vi "SaveSpe.vi"(0 "Live Time":dbl=1000.0, 1 "Z":dbl, 2 "Y":dbl, 3 "X":dbl, 4 "Real Time":dbl=1000.0, 5 "Spectrum":i32[](array[numeric]), 6 "name":string, 7 "data folder path":path) -> ()   [LabVIEW 2015]
panel:
  out "data size":i32
  out "error out 2":errorcluster
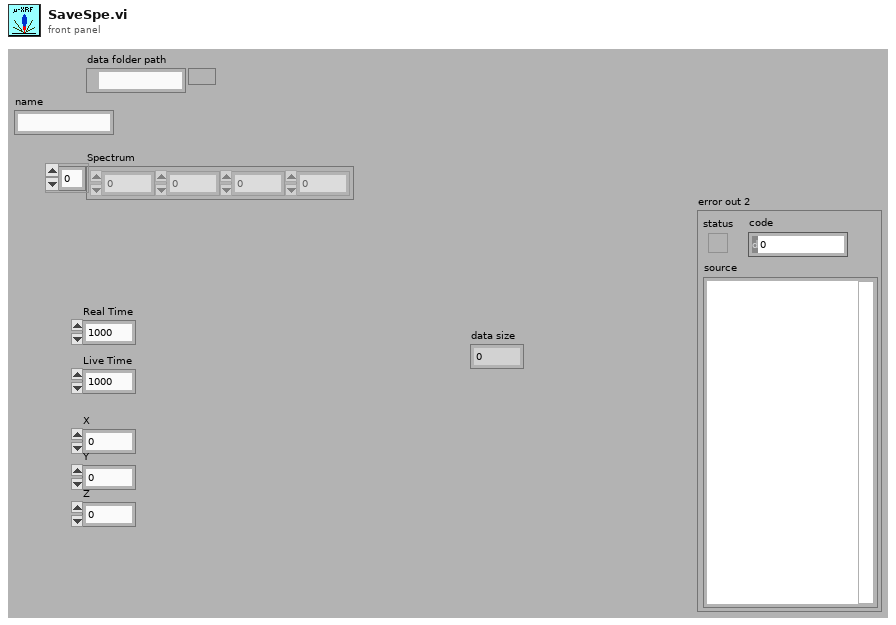
[diagram p1: front panel]
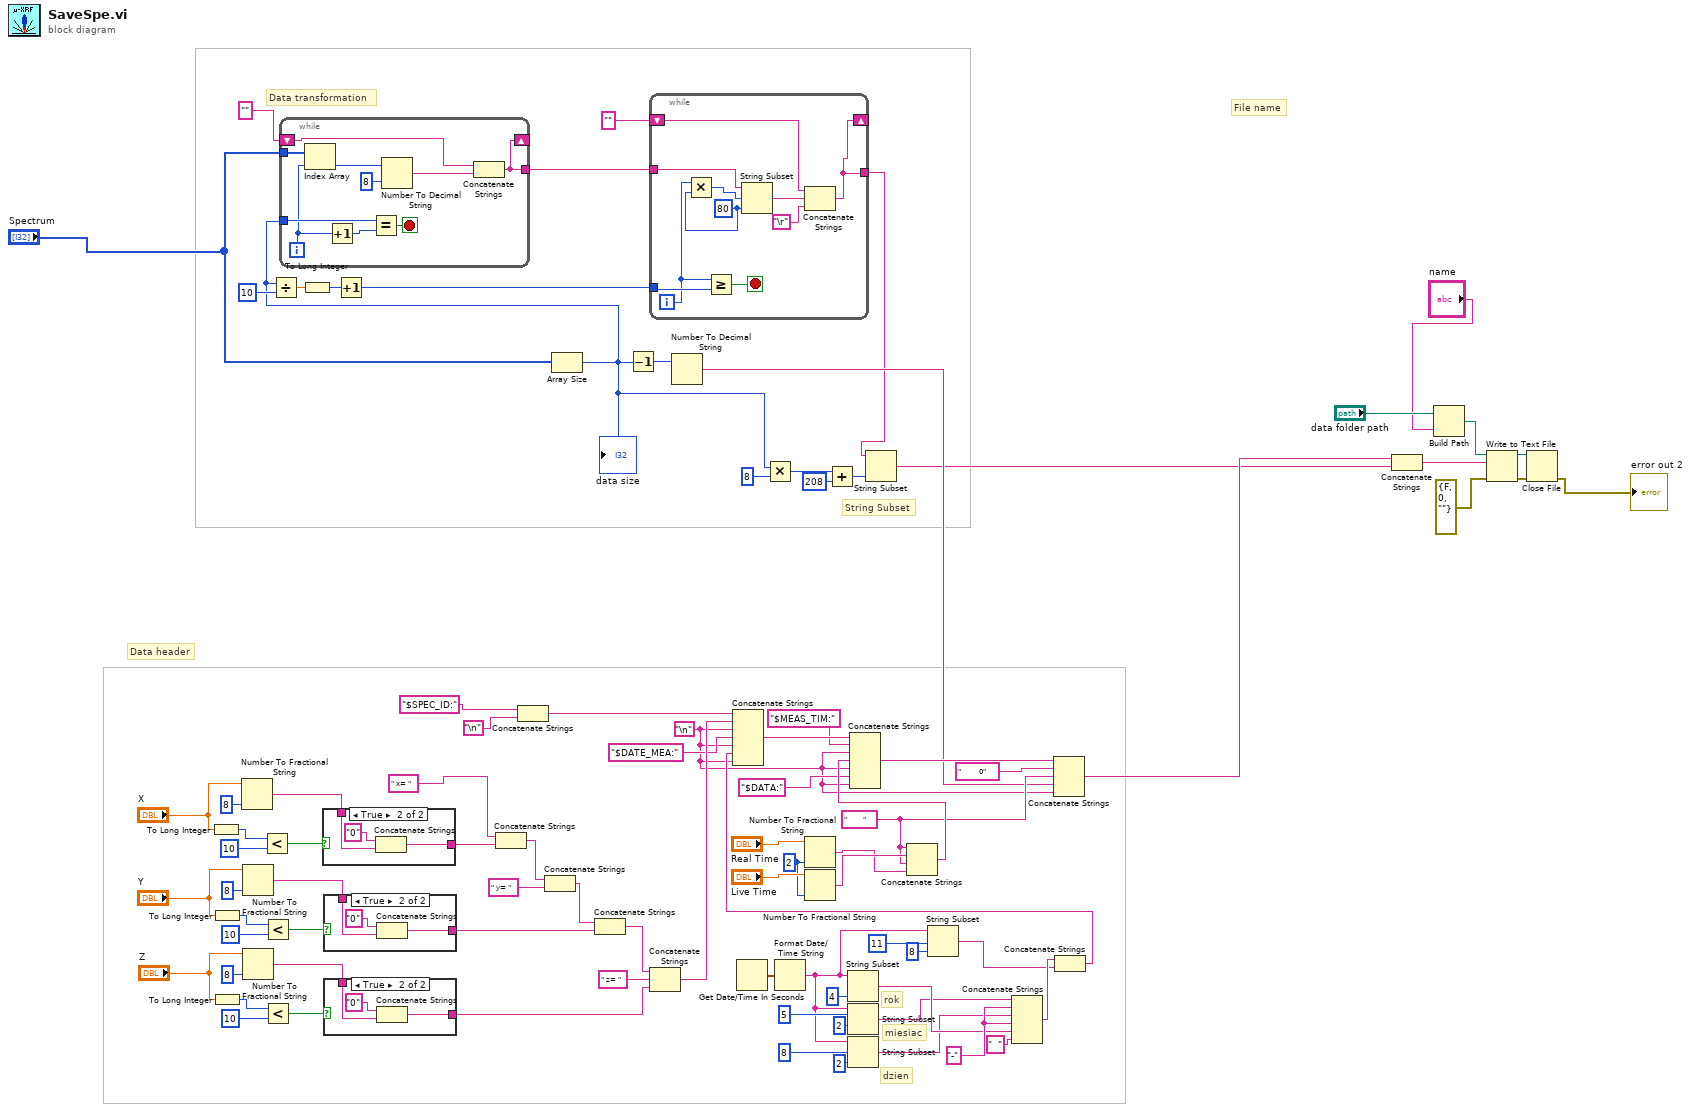
[diagram p0: block diagram]
diagram:
  w4 = i16 2 ("precision (6)")
  w29 = "        "
  w51 = "-"
  w27 = "\n"
  # "String Subset"
  # "Data transformation"
  # "Data header"
  # "File name"
  # "dzien"
  # "miesiac"
  # "rok"
  n1 = To Long Integer(number="X") -> (32bit integer=w83:i32)
  n2 = To Long Integer(number="Y") -> (32bit integer=w76:i32)
  n3 = To Long Integer(number="Z") -> (32bit integer=w69:i32)
  n4 = Number To Fractional String(number="X", precision (6)=i16 8) -> (F-format string=w84:string)  [unwired: 2 in]
  n5 = Number To Fractional String(number="Y", precision (6)=i16 8) -> (F-format string=w77:string)  [unwired: 2 in]
  n6 = Number To Fractional String(number="Z", precision (6)=i16 8) -> (F-format string=w70:string)  [unwired: 2 in]
  n7 = Less?(x=w83, y=10) -> (x < y?=w81:bool)
  n8 = Less?(x=w76, y=10) -> (x < y?=w74:bool)
  n9 = Less?(x=w69, y=10) -> (x < y?=w67:bool)
  n10 = case shown="True" w81 {
    tunnel: w84 -> [w89 w92]
    tunnel: [w89 w90] -> w79
    frame False {
    }
    frame True {
      n11 = Concatenate Strings("0" ("string"), w92) -> (w90:string)
    }
  }
  n12 = case shown="True" w74 {
    tunnel: w77 -> [w93 w96]
    tunnel: [w93 w94] -> w72
    frame False {
    }
    frame True {
      n13 = Concatenate Strings("0" ("string"), w96) -> (w94:string)
    }
  }
  n14 = case shown="True" w67 {
    tunnel: w70 -> [w97 w100]
    tunnel: [w97 w98] -> w63
    frame False {
    }
    frame True {
      n15 = Concatenate Strings("0" ("string"), w100) -> (w98:string)
    }
  }
  n16 = Concatenate Strings(" x= " ("string"), w79) -> (w88:string)
  n17 = Concatenate Strings("$SPEC_ID:", "\n") -> (w60:string)
  n18 = Concatenate Strings(w88, " y= " ("string")) -> (w86:string)
  n19 = Array Size(array="Spectrum") -> (size(s)=w16:i32)
  "data size" <- w16
  n20 = Divide(x=w16, y=10) -> (x/y=w25:dbl)
  n21 = while {
    tunnel: "Spectrum" -> [w108]
    tunnel: w16 -> [w107]
    tunnel: [w102] -> w22
    shift-right: [w102] -> _
    shift-left: "" -> [w101]
    i -> [w104]
    stop <- w106 stop-if-true
    n22 = Index Array(array=w108, index=w104) -> (element=w103:i32)
    n23 = Increment(x=w104) -> (x+1=w105:i32)
    n24 = Equal?(x=w107, y=w105) -> (x = y?=w106:bool)
    n25 = Number To Decimal String(number=w103, width (-)=i16 8) -> (decimal integer string=w109:string)
    n26 = Concatenate Strings(w101, w109) -> (w102:string)
  }
  n27 = To Long Integer(number=w25) -> (32bit integer=w24:i32)
  n28 = Increment(x=w24) -> (x+1=w23:i32)
  n29 = Concatenate Strings(w86, w72) -> (w65:string)
  n30 = Decrement(x=w16) -> (x-1=w32:i32)
  n31 = while {
    tunnel: w23 -> [w119]
    tunnel: w22 -> [w120]
    tunnel: [w112] -> w7
    shift-right: [w112] -> _
    shift-left: "" -> [w111]
    i -> [w115]
    stop <- w118 stop-if-true
    w116 = 80 ("length (rest)")
    n32 = Multiply(x=w115, y=w116) -> (x*y=w117:i32)
    n33 = Greater Or Equal?(x=w115, y=w119) -> (x >= y?=w118:bool)
    n34 = String Subset(string=w120, offset (0)=w117, length (rest)=w116) -> (substring=w114:string)
    n35 = Concatenate Strings(w111, w114, "\r") -> (w112:string)
  }
  n36 = Concatenate Strings(w65, " z= " ("string"), w63) -> (w59:string)
  n37 = Number To Decimal String(number=w32) -> (decimal integer string=w28:string)  [unwired: 1 in]
  n38 = Get Date/Time In Seconds() -> (seconds since 1Jan1904=w57:timestamp)
  n39 = Multiply(x=w16, y=8) -> (x*y=w14:i32)
  n40 = Format Date/Time String(seconds (now)=w57) -> (date/time string=w44:string)  [unwired: 2 in]
  n41 = Number To Fractional String(number="Real Time", precision (6)=w4) -> (F-format string=w35:string)  [unwired: 2 in]
  n42 = Number To Fractional String(number="Live Time", precision (6)=w4) -> (F-format string=w36:string)  [unwired: 2 in]
  n43 = Add(x=w14, y=208) -> (x+y=w9:i32)
  n44 = String Subset(string=w44, length (rest)=4 ("length (rest)")) -> (substring=w50:string)  [unwired: 1 in]
  n45 = String Subset(string=w44, offset (0)=5, length (rest)=2 ("length (rest)")) -> (substring=w43:string)
  n46 = String Subset(string=w44, offset (0)=8, length (rest)=2 ("length (rest)")) -> (substring=w42:string)
  n47 = String Subset(string=w7, length (rest)=w9) -> (substring=w8:string)  [unwired: 1 in]
  n48 = Concatenate Strings(w29, w36, w29, w35) -> (w34:string)
  n49 = String Subset(string=w44, offset (0)=11, length (rest)=8 ("length (rest)")) -> (substring=w45:string)
  n50 = Concatenate Strings(w43, w51, w42, w51, w50, "  " ("string")) -> (w46:string)
  n51 = Concatenate Strings(w46, w45) -> (w41:string)
  n52 = Concatenate Strings(w60, w59, w27, "$DATE_MEA:", w27, w41, w27) -> (w40:string)
  n53 = Concatenate Strings(w40, "$MEAS_TIM:", w27, w34, w27, "$DATA:" ("string"), w27) -> (w31:string)
  n54 = Concatenate Strings(w31, "         0" ("string"), w29, w28, w27) -> (w17:string)
  n55 = Concatenate Strings(w17, w8) -> (w18:string)
  n56 = Build Path(base path="data folder path", name or relative path="name") -> (appended path=w20:path)
  n57 = Write to Text File(file (use dialog)=w20, text=w18, error in=errorcluster {"status"=FALSE, "code"=0, "source"=""}) -> (refnum out=w12:refnum<file>, error out=w11:errorcluster)  [unwired: 1 in, 1 out]
  n58 = Close File(refnum=w12, error in=w11) -> (error out=→"error out 2":errorcluster)  [unwired: 1 out]
